vi "RollerSpeed_Contactor.vi"() -> ()   [LabVIEW 2019]
uses:
  <vilib>/Instr/_visa.llb/VISA Configure Serial Port (Instr).vi
panel:
  out "Current":sgl
  out "Voltage":sgl
  out "Speed Chart 2":dynamicdata(graph)
  out "Speed Chart":dynamicdata(graph)
  in  "t":sgl
  in  "test":bool
  out "WheelSpeed":sgl
  out "read buffer":string
  in  "?":bool
  out "RollerSpeed":sgl
  in  "VISA resource name":refnum<visa-resource-name>="COM5"
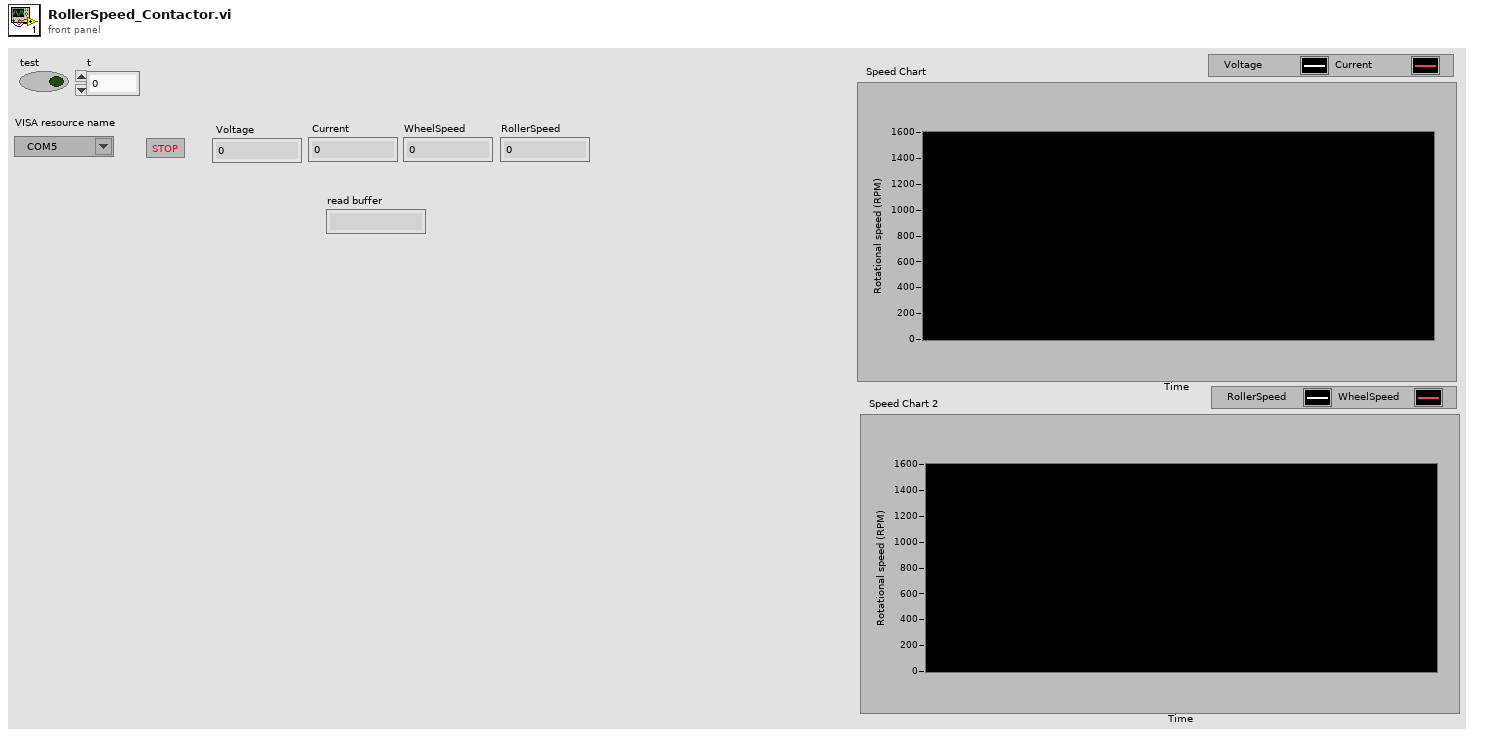
[diagram p1: front panel]
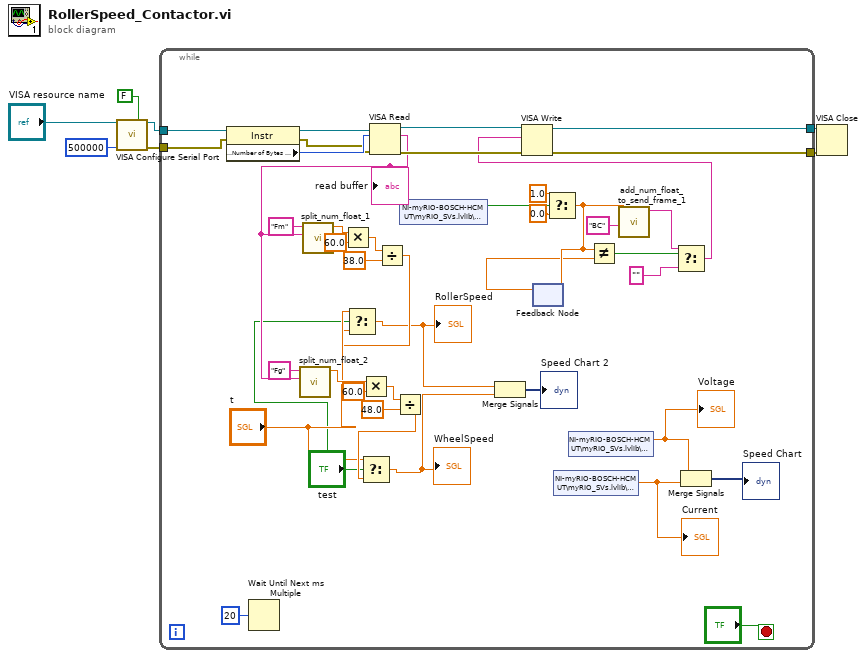
[diagram p0: block diagram]
diagram:
  n1 = call-poly "VISA Configure Serial Port"("VISA resource name"="VISA resource name", "Enable Termination\nChar (T)"=FALSE ("Enable Termination\nChar (T)"), "baud rate (9600)"=u32 500000) -> ("VISA resource name out"=w7:refnum<visa-resource-name>, "error out"=w6:errorcluster)  [unwired: 11 in]
  n2 = while {
    tunnel: w7 -> [w49]
    tunnel: w6 -> [w48]
    tunnel: [w42] -> w5
    tunnel: [w41] -> w4
    stop <- "?" stop-if-true
    n3 = property class="Instr"(reference=w49, error in=w48) -> (reference out=w47:refnum<visa-resource-name>, error out=w45:errorcluster, "Serial Settings:Number of Bytes at Serial Port"=w46:u32)
    n4 = Wait Until Next ms Multiple(millisecond multiple=u32 20) -> ()  [unwired: 1 out]
    n5 = VISA Read(VISA resource name=w47, byte count=w46, error in (no error)=w45) -> (VISA resource name out=w44:refnum<visa-resource-name>, read buffer=w18:string, error out=w43:errorcluster)  [unwired: 1 out]
    "read buffer" <- w18
    n6 = call "split_num_float_2.vi"("read_frame"=w18, "id (2 characters)"="Fg") -> ("num_float"=w20:sgl)  [unwired: 9 in]
    n7 = call "split_num_float_1.vi"("read_frame"=w18, "id (2 characters)"="Fm") -> ("num_float"=w35:sgl)  [unwired: 9 in]
    n8 = Multiply(x=w35, y=sgl 60.0) -> (x*y=w36:sgl)
    n9 = Multiply(x=w20, y=sgl 60.0) -> (x*y=w21:sgl)
    n10 = Divide(x=w36, y=sgl 38.0) -> (x/y=w15:sgl)
    n11 = Select(t="t", s="test", f=w15) -> (s? t:f=w11:sgl)
    "RollerSpeed" <- w11
    n12 = Divide(x=w21, y=sgl 48.0) -> (x/y=w17:sgl)
    n13 = Select(t="t", s="test", f=w17) -> (s? t:f=w10:sgl)
    "WheelSpeed" <- w10
    n14 = shared-variable "NI-myRIO-BOSCH-HCMUT\\myRIO_SVs.lvlib\\Boolean"() -> (w27:bool)  [unwired: 1 in, 1 out]
    n15 = Merge Signals(w11, w10) -> (→"Speed Chart 2":dynamicdata)
    n16 = feedback #1() -> (w24:sgl)  [unwired: 1 in]
    n17 = Select(t=sgl 1.0, s=w27, f=sgl 0.0) -> (s? t:f=w25:sgl)
    n18 = feedback-in #1(w25) -> ()
    n19 = shared-variable "NI-myRIO-BOSCH-HCMUT\\myRIO_SVs.lvlib\\Current"() -> (w8:dbl)  [unwired: 1 in, 1 out]
    "Current" <- w8
    n20 = shared-variable "NI-myRIO-BOSCH-HCMUT\\myRIO_SVs.lvlib\\Voltage"() -> (w9:dbl)  [unwired: 1 in, 1 out]
    "Voltage" <- w9
    n21 = Not Equal?(x=w25, y=w24) -> (x != y?=w26:bool)
    n22 = call "add_num_float_to_send_frame_1.vi"("num_float"=w25, "id (2 characters)"="BC") -> ("String"=w40:string)  [unwired: 9 in]
    n23 = Select(t=w40, s=w26, f="") -> (s? t:f=w39:string)
    n24 = VISA Write(VISA resource name=w44, write buffer=w39, error in (no error)=w43) -> (VISA resource name out=w41:refnum<visa-resource-name>, error out=w42:errorcluster)  [unwired: 1 out]
    n25 = Merge Signals(w9, w8) -> (→"Speed Chart":dynamicdata)
  }
  n26 = VISA Close(VISA resource name=w4, error in (no error)=w5) -> ()  [unwired: 1 out]
